vi "PumpGame.vi"() -> ()   [LabVIEW 2020]
doc: "Simple game, examplary of producer/consumer architecture. Comments in Polish."
panel:
  out "Score":string="Score:0"
  in  "Pump":bool
  out "Tank":dbl(slide)=100.0 scale=0.0..100.0
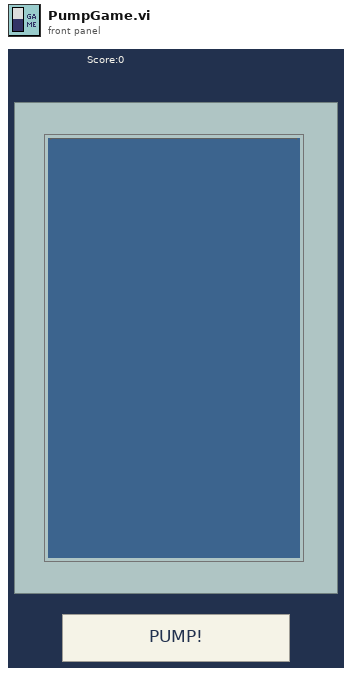
[diagram p1: front panel]
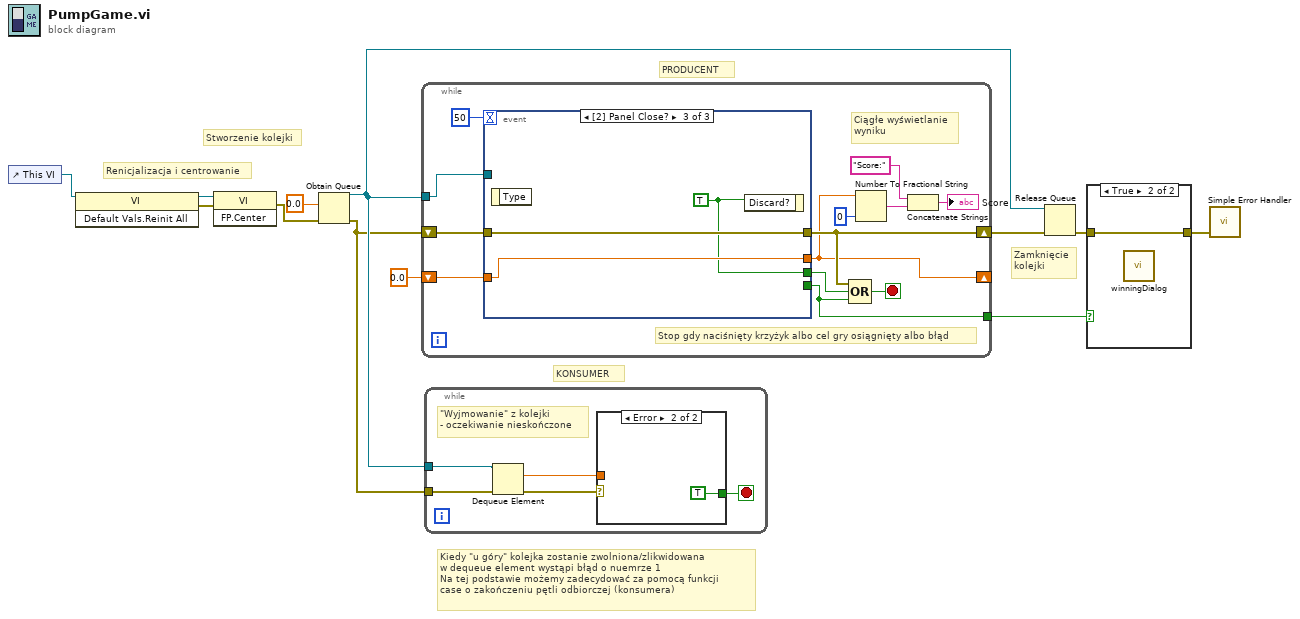
[diagram p0: block diagram]
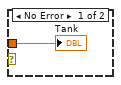
[diagram p3: hidden frame]
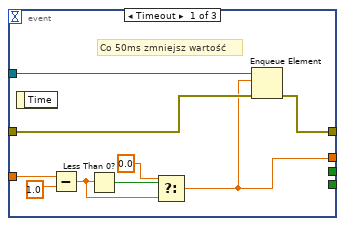
[diagram p4: hidden frame]
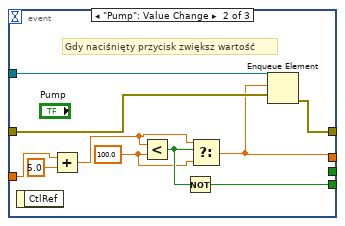
[diagram p5: hidden frame]
diagram:
  # "Zamknięcie\nkolejki"
  # "PRODUCENT"
  # "KONSUMER"
  # "Renicjalizacja i centrowanie"
  # "Kiedy \"u góry\" kolejka zostanie zwolniona/zlikwidowana\nw dequeue element wystąpi błąd o nuemrze 1 \nNa tej podstawie możemy zadecydować za pomocą funkcji \ncase o zakończeniu pętli odbiorczej (konsumera)"
  # "Stworzenie kolejki"
  n1 = control-ref of="This VI"() -> (w4:refnum<vi>)
  n2 = invoke class="VI" method="Default Vals.Reinit All"(reference=w4) -> (reference out=w3:refnum<vi>, error out=w2:errorcluster)  [unwired: 2 in, 1 out]
  n3 = invoke class="VI" method="FP.Center"(reference=w3, error in=w2) -> (error out=w1:errorcluster)  [unwired: 1 in, 2 out]
  n4 = Obtain Queue(element data type=0.0, error in (no error)=w1) -> (queue out=w10:refnum<queue>, error out=w9:errorcluster)  [unwired: 3 in, 1 out]
  n5 = while {
    shift-right: [w22] -> w11
    shift-left: w9 -> [w25]
    tunnel: w10 -> [w23]
    shift-right: [w18] -> _
    shift-left: 0.0 -> [w20]
    tunnel: [w19] -> w7
    stop <- w21 stop-if-true
    # "Ciągłe wyświetlanie\nwyniku"
    # "Stop gdy naciśnięty krzyżyk albo cel gry osiągnięty albo błąd"
    n6 = event shown="[2] Panel Close?" {
      selector: _ -> [_ _ _]
      dyn-events: _ -> [_ _ _]
      timeout: 50 -> [_ _ _]
      tunnel: w25 -> [w33 w43 w47]
      tunnel: [w34 w44 w47] -> w22
      tunnel: w23 -> [w32 w42 _]
      tunnel: w20 -> [w31 w41 w46]
      tunnel: [_ w35 _] -> w19
      tunnel: [w27 w36 w46] -> w18
      tunnel: [_ _ w45] -> w15
      event Timeout {
        # "Co 50ms zmniejsz wartość"
        n7 = event-data() -> ()  [unwired: 1 in, 1 out]
        n8 = Subtract(x=w31, y=1.0) -> (x-y=w28:dbl)
        n9 = Less Than 0?(x=w28) -> (x < 0?=w26:bool)
        n10 = Select(t=0.0, s=w26, f=w28) -> (s? t:f=w27:dbl)
        n11 = Enqueue Element(queue=w32, element=w27, error in (no error)=w33) -> (error out=w34:errorcluster)  [unwired: 1 in, 2 out]
      }
      event "Pump": Value Change {
        w37 = 100.0 ("y")
        # "Gdy naciśnięty przycisk zwiększ wartość"
        n12 = event-data() -> ()  [unwired: 1 in, 1 out]
        n13 = Add(x=w41, y=5.0) -> (x+y=w38:dbl)
        n14 = Less?(x=w38, y=w37) -> (x < y?=w39:bool)
        n15 = Not(x=w39) -> (.not. x?=w35:bool)
        n16 = Select(t=w38, s=w39, f=w37) -> (s? t:f=w36:dbl)
        n17 = Enqueue Element(queue=w42, element=w36, error in (no error)=w43) -> (error out=w44:errorcluster)  [unwired: 1 in, 2 out]
      }
      event Panel Close? {
        w45 = TRUE
        n18 = event-data() -> ()  [unwired: 1 in, 1 out]
        n19 = event-data("Discard?"=w45) -> ()  [unwired: 1 in, 1 out]
      }
    }
    n20 = Compound Arithmetic op=OR(w22, w15, w19) -> (w21:bool)
    n21 = Number To Fractional String(number=w18, precision (6)=i16 0) -> (F-format string=w17:string)  [unwired: 2 in]
    n22 = Concatenate Strings("Score:" ("string"), w17) -> (→"Score":string)
  }
  n23 = while {
    tunnel: w10 -> [w52]
    tunnel: w9 -> [w48]
    stop <- w49 stop-if-true
    # "\"Wyjmowanie\" z kolejki\n- oczekiwanie nieskończone"
    n24 = Dequeue Element(queue=w52, error in (no error)=w48) -> (element=w51:dbl, error out=w50:errorcluster)  [unwired: 1 in, 2 out]
    n25 = case shown="Error" w50 {
      tunnel: w51 -> [w53 _]
      tunnel: [_ TRUE] -> w49
      frame No Error {
        "Tank" <- w53
      }
      frame Error {
      }
    }
  }
  n26 = Release Queue(queue=w10, error in (no error)=w11) -> (error out=w6:errorcluster)  [unwired: 1 in, 2 out]
  n27 = case shown="True" w7 {
    tunnel: w6 -> [w55 w56]
    tunnel: [w55 w56] -> w5
    frame False {
    }
    frame True {
      n28 = call "winningDialog.vi"() -> ()  [unwired: 1 in]
    }
  }
  n29 = call <vilib>:"Simple Error Handler.vi"("error in (no error)"=w5) -> ()  [unwired: 4 in, 5 out]
